vi "Copy Node.vi"(7 "New Parent Path in Target":string, 8 "Remove (False)":bool, 9 "Source Tree Map (Use Target)":T1, 10 "Node Path in Source":string, 11 "Target Tree Map In":T1) -> (0 "Path Invalid":bool, 3 "Target Tree Map Out":T1, 5 "New Paths":set{string}(c389))   [LabVIEW 2019, in "Tree Map.lvlib"]
doc: "Make a copy of a node specified by path. In order to move a node the optional Remove flag can be set to True.\n\nYou can optionally specify a different Tree Map as the source of the node to copy. If you leave the input unwired the Target Tree Map will be used both as Source and Target. Using this option you can copy segments of one Tree Map into another Tree Map.\n\n<b>Author:</b> Piotr Kruczkowski <PrimaryKey>\n<b>License:</b> NewBSD\n\nCopyright (c) 2019, National Instruments\nAll rights reserved.\n\nRedistribution and use in source and binary forms, with or without\nmodification, are permitted provided that the following conditions are met:\n1. Redistributions of source code must retain the above copyright\n notice, this list of conditions and the following disclaimer.\n2. Redistributions in binary form must reproduce the above copyright\n notice, this list of conditions and the following disclaimer in the\n documentation and/or other materials provided with the distribution.\n3. Neither the name of National Instruments nor the\n names of its contributors may be used to endorse or promote products\n derived from this software without specific prior written permission.\n\nTHIS SOFTWARE IS PROVIDED BY National Instruments ''AS IS'' AND ANY\nEXPRESS OR IMPLIED WARRANTIES, INCLUDING, BUT NOT LIMITED TO, THE IMPLIED\nWARRANTIES OF MERCHANTABILITY AND FITNESS FOR A PARTICULAR PURPOSE ARE\nDISCLAIMED. IN NO EVENT SHALL National Instruments BE LIABLE FOR ANY\nDIRECT, INDIRECT, INCIDENTAL, SPECIAL, EXEMPLARY, OR CONSEQUENTIAL DAMAGES\n(INCLUDING, BUT NOT LIMITED TO, PROCUREMENT OF SUBSTITUTE GOODS OR SERVICES;\nLOSS OF USE, DATA, OR PROFITS; OR BUSINESS INTERRUPTION) HOWEVER CAUSED AND\nON ANY THEORY OF LIABILITY, WHETHER IN CONTRACT, STRICT LIABILITY, OR TORT\n(INCLUDING NEGLIGENCE OR OTHERWISE) ARISING IN ANY WAY OUT OF THE USE OF THIS\nSOFTWARE, EVEN IF ADVISED OF THE POSSIBILITY OF SUCH DAMAGE."
uses:
  Tree Map.lvlib
  Tree Map Data.ctl
  c8bc83a8-2c75-448f-9bd4-d78f320d1bbe.vi
  Utility/Get Parent Path.vi/c149eb16-3742-4982-a86f-30a3e2ff274e.vi
  Utility/Join Strings Tree.vi
  Utility/Get Parent Path.vi/818a8d1e-6665-467f-8da4-62c25be60167.vi
  Utility/Split String Tree.vi
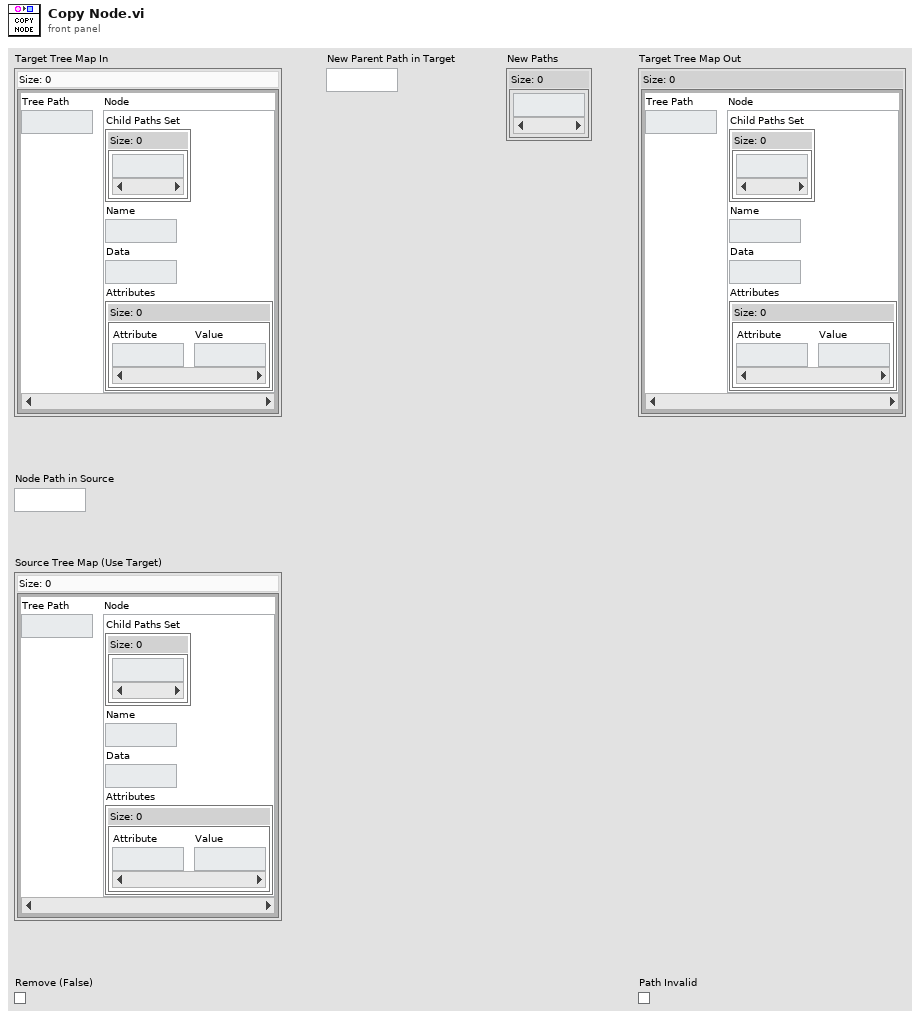
[diagram p1: front panel]
types:
  T1 = typedef "Tree Map.lvlib/Tree Map Data.ctl" = map{string, cluster{"Child Paths Set":set{string}, "Name":string, "Data":string, "Attributes":map{string, string}}}
  T2 = cluster{"Child Paths Set":set{string}, "Name":string, "Data":string, "Attributes":map{string, string}}
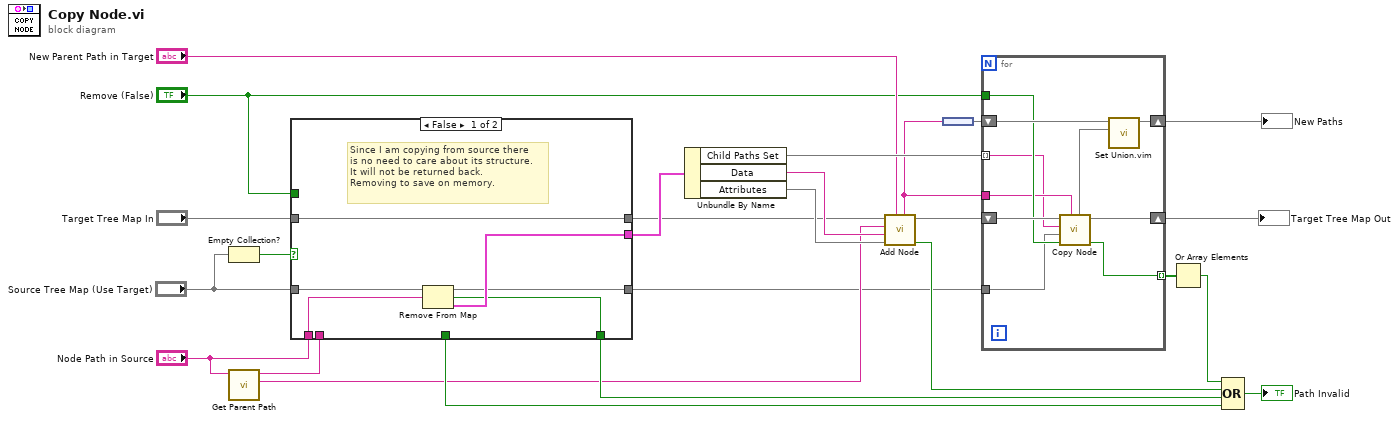
[diagram p0: block diagram]
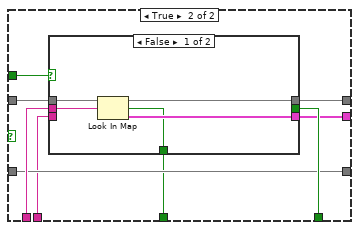
[diagram p2: hidden frame]
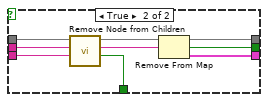
[diagram p3: hidden frame]
diagram:
  n1 = Empty Collection?(1:"Source Tree Map (Use Target)") -> (0:w4:bool)
  n2 = call "Get Parent Path.vi"("Node Path"="Node Path in Source") -> ("Node Name"=w9:string, "Parent Path"=w7:string)  [unwired: 8 in, 1 out]
  n3 = case shown="False" w4 {
    tunnel: [w29 w40] -> w22
    tunnel: [_ w33] -> w21
    tunnel: [w30 w39] -> w17
    tunnel: "Remove (False)" -> [_ w32]
    tunnel: w7 -> [_ w35]
    tunnel: "Node Path in Source" -> [w31 w38]
    tunnel: "Target Tree Map In" -> [w28 w34]
    tunnel: "Source Tree Map (Use Target)" -> [w27 w37]
    tunnel: [w26 w37] -> w2
    tunnel: [w28 w36] -> w1
    frame False {
      # "Since I am copying from source there\nis no need to care about its structure.\nIt will not be returned back. \nRemoving to save on memory."
      n4 = Remove From Map(10:w31, 11:w27) -> (1:w30:T2, 2:w29:bool, 3:w26:T1)
    }
    frame True {
      n5 = case shown="False" w32 {
        tunnel: w38 -> [w44 w48]
        tunnel: [w42 w52] -> w36
        tunnel: [w43 w51] -> w39
        tunnel: [_ w50] -> w40
        tunnel: w35 -> [_ w49]
        tunnel: w34 -> [w42 w47]
        tunnel: [w41 w46] -> w33
        frame False {
          n6 = Look In Map(map=w42, key=w44) -> (key not found?=w41:bool, value=w43:T2)  [unwired: 1 in]
        }
        frame True {
          n7 = call "Remove Node from Children.vi"("Parent Path"=w49, "Node Path In"=w48, "Tree Map In"=w47) -> ("Path Invalid"=w46:bool, "Tree Map Out"=w45:T1)  [unwired: 7 in]
          n8 = Remove From Map(10:w48, 11:w45) -> (1:w51:T2, 2:w50:bool, 3:w52:T1)
        }
      }
    }
  }
  n9 = Unbundle By Name(w17) -> ("Child Paths Set"=w16:set{string}, "Data"=w12:string, "Attributes"=w11:map{string, string})
  n10 = call "Add Node.vi"("Parent Path"="New Parent Path in Target", "Attributes"=w11, "Data"=w12, "New Node Name"=w9, "Tree Map In"=w1) -> ("Path Invalid"=w10:bool, "Tree Map Out"=w25:T1, "New Node Path"=w13:string)  [unwired: 4 in]
  n11 = node(w13) -> (w24:set{string})
  n12 = for {
    shift-right: [w61] -> w15
    shift-left: w25 -> [w62]
    shift-right: [w59] -> w23
    shift-left: w24 -> [w60]
    tunnel: w13 -> [w54]
    tunnel: w16 -> [w53] mode=indexing
    tunnel: [w57] -> w19 mode=indexing
    tunnel: "Remove (False)" -> [w56]
    tunnel: w2 -> [w55]
    n13 = call "Copy Node.vi"("New Parent Path in Target"=w54, "Remove (False)"=w56, "Source Tree Map (Use Target)"=w55, "Node Path in Source"=w53, "Target Tree Map In"=w62) -> ("Path Invalid"=w57:bool, "Target Tree Map Out"=w61:T1, "New Paths"=w58:set{string})  [unwired: 4 in]
    n14 = call "Set Union.vim"("set 2"=w58, "set 1"=w60) -> ("union"=w59:set{string})  [unwired: 9 in]
  }
  "New Paths" <- w23
  "Target Tree Map Out" <- w15
  n15 = Or Array Elements(Boolean array=w19) -> (logical OR=w18:bool)
  n16 = Compound Arithmetic op=OR(w18, w10, w22, w21) -> (→"Path Invalid":bool)
